vi "Get Type.vi"(8 "error in (no error)":errorcluster, 11 "Device in":refnum<class "Device.lvclass">) -> (0 "error out":errorcluster, 2 "Type":string, 3 "Device out":refnum<class "Device.lvclass">)   [LabVIEW 2020, in "HAL.lvlib" / "Device.lvclass"]
doc: "Intermediate device type classes need to override this VI to provide the device type for editors. Type can be values such as Power Supply, DUT, Camera, etc. and represent a group of devices that perform the same collection of actions. For instance, most power supplies provide the ability to turn on or off the output, set voltage, measure current, and measure actual voltage."
uses:
  Device.lvclass
  <vilib>/Utility/error.llb/Error Cluster From Error Code.vi
  <vilib>/ErrorRing/Error Ring.xnode
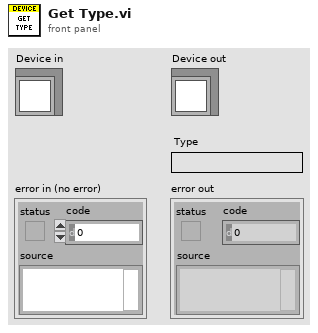
[diagram p1: front panel]
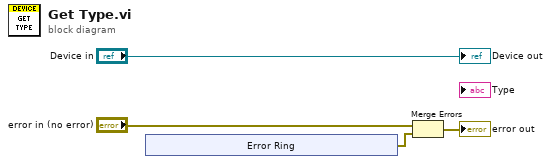
[diagram p0: block diagram]
diagram:
  n1 = xnode "Error Ring"() -> ("error out"=w1:errorcluster)
  n2 = Merge Errors("error in (no error)", w1) -> (→"error out":errorcluster)
  "Device out" <- "Device in"
